vi "Calculate Distance.vi"(4 "Prime Meridian Destination Direction":string, 5 "Equator Destination Direction":string, 6 "Destination Longitude":dbl, 7 "Destination Latitude":dbl, 8 "East or West":string, 9 "Longitude":dbl, 10 "North or South":string, 11 "Latitude":dbl) -> (3 "Distance (ft)":dbl)   [LabVIEW 2011]
uses:
  <vilib>/express/express arith-compare/Formula/XNode/ExpressFormulaBlockNode.xnode
panel:
  out "CurLongRad":dbl
  out "CurLatRad":dbl
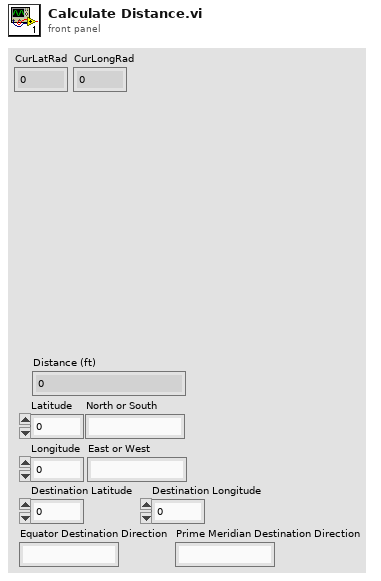
[diagram p1: front panel]
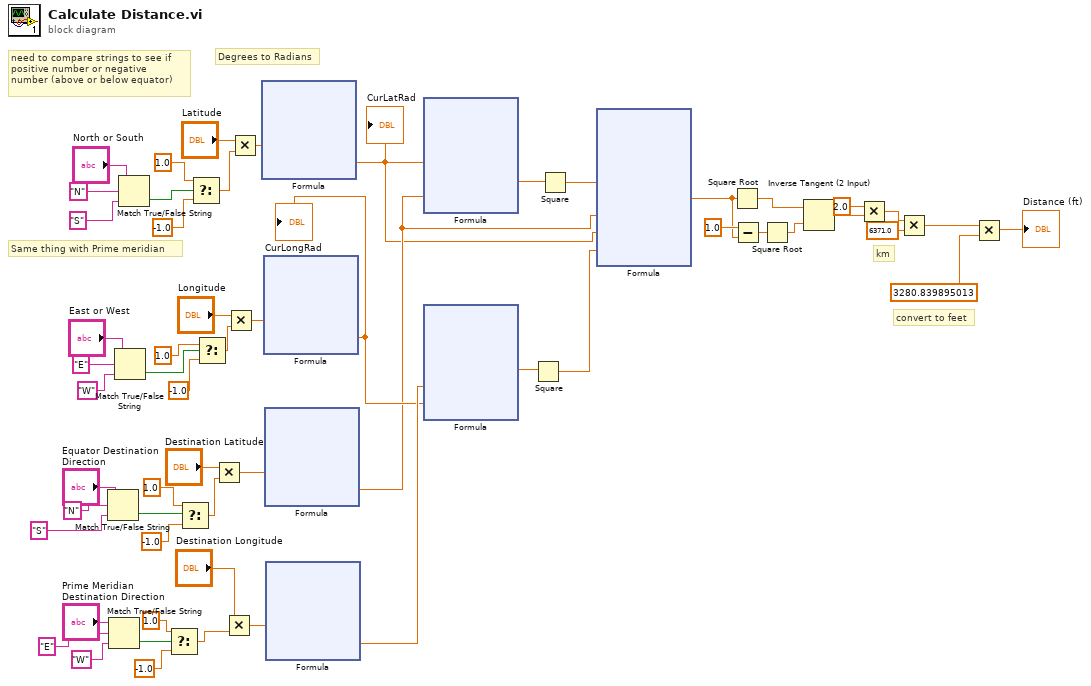
[diagram p0: block diagram]
diagram:
  # "convert to feet"
  # "km"
  # "Same thing with Prime meridian"
  # "need to compare strings to see if \npositive number or negative \nnumber (above or below equator)"
  # "Degrees to Radians"
  n1 = Match True/False String(2:"S" ("false string"), 3:"N" ("true string"), 4:"Equator Destination Direction") -> (0:w53:bool)  [unwired: 1 out]
  n2 = Match True/False String(2:"W" ("false string"), 3:"E" ("true string"), 4:"Prime Meridian Destination Direction") -> (0:w45:bool)  [unwired: 1 out]
  n3 = Match True/False String(2:"W" ("false string"), 3:"E" ("true string"), 4:"East or West") -> (0:w36:bool)  [unwired: 1 out]
  n4 = Match True/False String(2:"S" ("false string"), 3:"N" ("true string"), 4:"North or South") -> (0:w33:bool)  [unwired: 1 out]
  n5 = Select(t=1.0, s=w45, f=-1.0) -> (s? t:f=w55:dbl)
  n6 = Select(t=1.0, s=w53, f=-1.0) -> (s? t:f=w54:dbl)
  n7 = Select(t=1.0, s=w33, f=-1.0) -> (s? t:f=w40:dbl)
  n8 = Select(t=1.0, s=w36, f=-1.0) -> (s? t:f=w39:dbl)
  n9 = Multiply(x="Destination Latitude", y=w54) -> (x*y=w44:dbl)
  n10 = Multiply(x="Destination Longitude", y=w55) -> (x*y=w43:dbl)
  n11 = Multiply(x="Longitude", y=w39) -> (x*y=w41:dbl)
  n12 = Multiply(x="Latitude", y=w40) -> (x*y=w42:dbl)
  n13 = xnode "Formula"("Dlat1"=w42) -> ("Result"=w13:dbl)  [unwired: 1 in, 1 out]
  "CurLatRad" <- w13
  n14 = xnode "Formula"("Dlong1"=w41) -> ("Result"=w18:dbl)  [unwired: 1 in, 1 out]
  "CurLongRad" <- w18
  n15 = xnode "Formula"("Dlat2"=w44) -> ("Result"=w14:dbl)  [unwired: 1 in, 1 out]
  n16 = xnode "Formula"("Dlong2"=w43) -> ("Result"=w19:dbl)  [unwired: 1 in, 1 out]
  n17 = xnode "Formula"("CurLatRad"=w13, "DesLatRad"=w14) -> ("Result"=w20:dbl)  [unwired: 1 in, 1 out]
  n18 = xnode "Formula"("DesLongRad"=w19, "CurLongRad"=w18) -> ("Result"=w17:dbl)  [unwired: 1 in, 1 out]
  n19 = Square(x=w17) -> (x^2=w16:dbl)
  n20 = Square(x=w20) -> (x^2=w15:dbl)
  n21 = xnode "Formula"("Part1"=w15, "DesLatRad"=w14, "CurLatRad"=w13, "Part2"=w16) -> ("Result"=w11:dbl)  [unwired: 1 in, 1 out]
  n22 = Square Root(x=w11) -> (sqrt(x)=w10:dbl)
  n23 = Subtract(x=1.0, y=w11) -> (x-y=w9:dbl)
  n24 = Square Root(x=w9) -> (sqrt(x)=w3:dbl)
  n25 = Inverse Tangent (2 Input)(1:w3, 2:w10) -> (0:w8:dbl)
  n26 = Multiply(x=2.0, y=w8) -> (x*y=w6:dbl)
  n27 = Multiply(x=w6, y=6371.0) -> (x*y=w4:dbl)
  n28 = Multiply(x=w4, y=3280.839895013) -> (x*y=→"Distance (ft)":dbl)
